vi "oax_Generate Piecewise Signal.vi"(4 "acc transition ratio":dbl=0.1, 6 "order":dbl, 7 "fs":dbl, 8 "init phase":dbl, 9 "time period":dbl, 10 "end speed":dbl, 11 "start speed/constant speed":dbl) -> (0 "final phase":dbl, 3 "phase out":dbl[](array[numeric]))   [LabVIEW 2017]
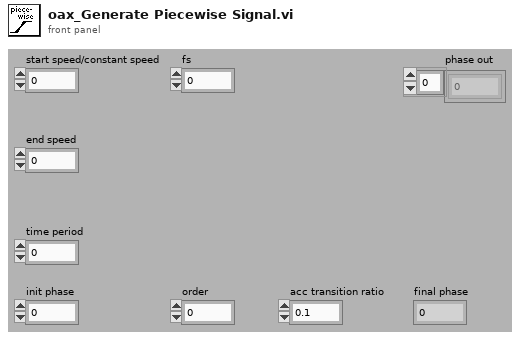
[diagram p1: front panel]
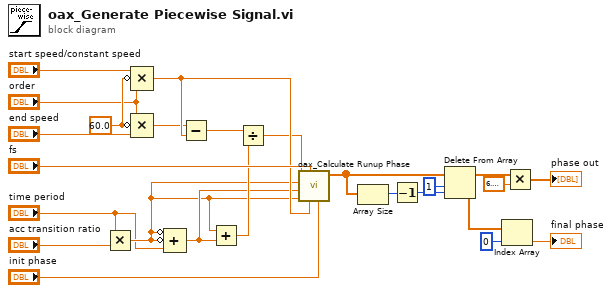
[diagram p0: block diagram]
diagram:
  w23 = 60.0 ("y")
  n1 = Multiply(x="time period", y="acc transition ratio") -> (x*y=w2:dbl)
  n2 = Compound Arithmetic op=MULTIPLY("start speed/constant speed", invert w23, "order") -> (w20:dbl)
  n3 = Compound Arithmetic op=MULTIPLY("order", invert w23, "end speed") -> (w19:dbl)
  n4 = Compound Arithmetic op=ADD(invert w2, invert w2, "time period") -> (w3:dbl)
  n5 = Subtract(x=w19, y=w20) -> (x-y=w15:dbl)
  n6 = Add(x=w2, y=w3) -> (x+y=w14:dbl)
  n7 = Divide(x=w15, y=w14) -> (x/y=w13:dbl)
  n8 = call <vilib>:"oax_Calculate Runup Phase.vi"("init phase"="init phase", "start freq"=w20, "fs"="fs", "post time period"=w2, "middle time period"=w3, "pre time period"=w2, "a"=w13) -> ("phase out"=w6:dbl[])  [unwired: 4 in]
  n9 = Array Size(array=w6) -> (size(s)=w8:i32)
  n10 = Decrement(x=w8) -> (x-1=w7:i32)
  n11 = Delete From Array(array=w6, length=1, index=w7) -> (deleted portion=w11:dbl[], array with subset deleted=w5:dbl[])
  n12 = Index Array(array=w11, index=0) -> (element=→"final phase":dbl)
  n13 = Multiply(x=w5, y=6.283185307179586) -> (x*y=→"phase out":dbl[])
